vi "setConfiguration.vi"(8 "error in (no error)":errorcluster, 10 "configuration":T1={"exposure_time_s"=nan, "delay_time_s"=nan, "roi"={"x0"=18446744073709551615, "y0"=18446744073709551615, "x1"=18446744073709551615, "y1"=18446744073709551615}, "timestamp_mode"=65535, "pixelrate"=4294967295, "trigger_mode"=65535, "acquire_mode"=65535, "metadata_mode"=65535, "noisefilter_mode"=65535, "binning"={"vert"=65535, "horz"=65535}} {"noisefilter_mode" items=["Undefined"=65535, "OFF"=0, "ON"=1]; "exposure_time_s" format="%#_6f"; "timestamp_mode" items=["Undefined"=65535, "OFF"=0, "Binary"=1, "Binary+ASCII"=2, "ASCII"=3]; "acquire_mode" items=["Undefined"=65535, "auto"=0, "external"=1, "external modulate"=2]; "trigger_mode" items=["Undefined"=65535, "auto sequence"=0, "software trigger"=1, "external exposure start & software trigger"=2, "external exposure control"=3, "external synchronized"=4, "fast external exposure control"=5, "external CDS control"=6, "slow external exposure control"=7, "external synchronized HDSDI"=258]; "metadata_mode" items=["Undefined"=65535, "OFF"=0, "ON"=1]}, 11 "Camera in":refnum<class "Camera.lvclass">) -> (0 "error out":errorcluster, 3 "Camera out":refnum<class "Camera.lvclass">)   [LabVIEW 2020, in "Camera.lvclass"]
doc: "Sets a new coniguration to the camera."
uses:
  Camera.lvclass
  Camera.lvclass/Camera.ctl
  TimingControl.lvlib
  ImageSensor.lvlib
  RecordingControl.lvlib
  GeneralCameraControl.lvlib
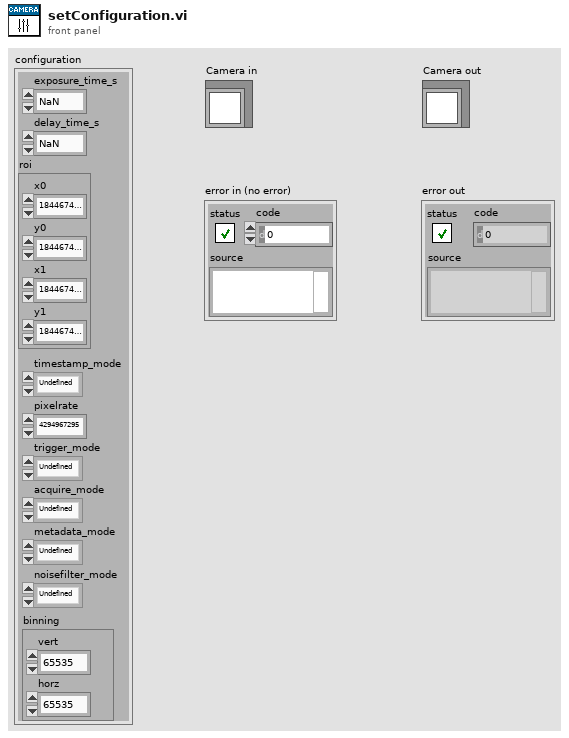
[diagram p1: front panel]
types:
  T1 = cluster{"exposure_time_s":dbl, "delay_time_s":dbl, "roi":cluster{"x0":u64, "y0":u64, "x1":u64, "y1":u64}, "timestamp_mode":u16, "pixelrate":u32, "trigger_mode":u16, "acquire_mode":u16, "metadata_mode":u16, "noisefilter_mode":u16, "binning":cluster{"vert":u16, "horz":u16}}
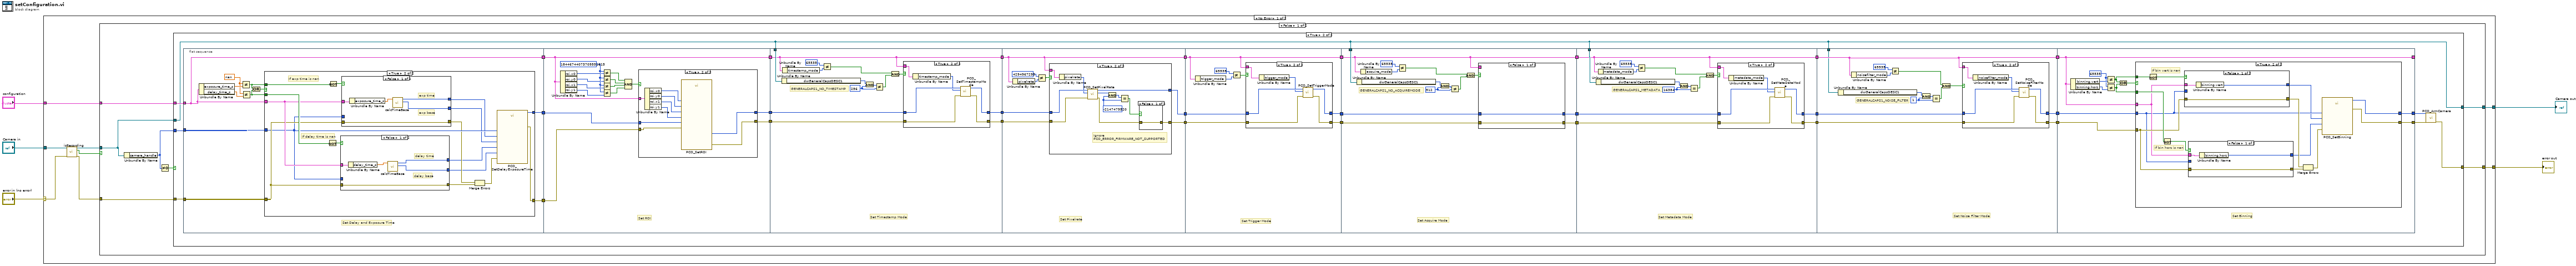
[diagram p0: block diagram]
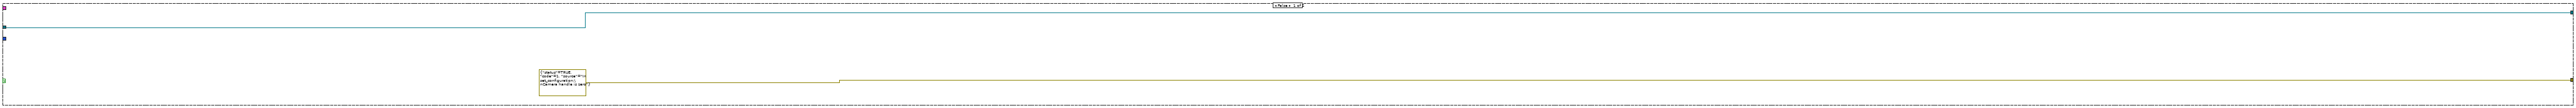
[diagram p2: hidden frame]
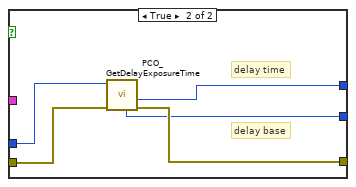
[diagram p4: hidden frame]
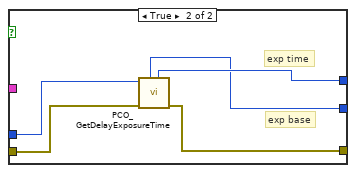
[diagram p5: hidden frame]
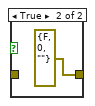
[diagram p9: hidden frame]
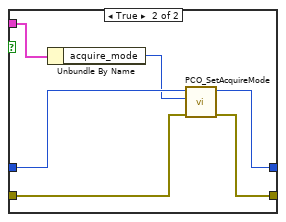
[diagram p11: hidden frame]
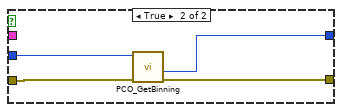
[diagram p15: hidden frame]
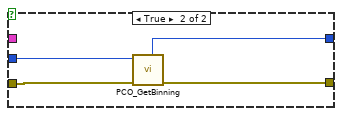
[diagram p16: hidden frame]
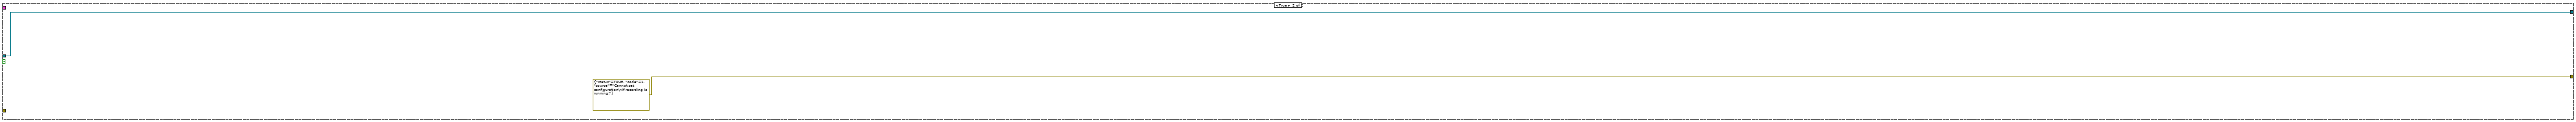
[diagram p17: hidden frame]
diagram:
  n1 = case shown="No Error" "error in (no error)" {
    selector: "error in (no error)" -> [w10 w300]
    tunnel: [w13 w300] -> w4
    tunnel: [w12 w299] -> w2
    tunnel: "Camera in" -> [w11 w299]
    tunnel: "configuration" -> [w6 _]
    frame No Error {
      n2 = call-dynamic "isRecording.vi"("Camera in"=w11, "error in (no error)"=w10) -> ("Camera out"=w7:refnum<class "Camera.lvclass">, "recording"=w9:bool, "error out"=w8:errorcluster)  [unwired: 11 in]
      n3 = case shown="False" w9 {
        tunnel: [w18 errorcluster {"status"=TRUE, "code"=1, "source"="Cannot set configuration\nif recording is running!"} ("error constant")] -> w13
        tunnel: [w17 w297] -> w12
        tunnel: w8 -> [w16 _]
        tunnel: w7 -> [w14 w297]
        tunnel: w6 -> [w15 _]
        frame False {
          n4 = Unbundle By Name(w14) -> ("camera_handle"=w19:u64)
          n5 = Not Equal To 0?(x=w19) -> (x != 0?=w20:bool)
          n6 = case shown="True" w20 {
            tunnel: [errorcluster {"status"=TRUE, "code"=1, "source"="In set_configuration:\nCamera handle is zero"} ("error constant") w24] -> w18
            tunnel: w19 -> [_ w53]
            tunnel: w16 -> [_ w52]
            tunnel: w14 -> [w21 w23]
            tunnel: [w21 w23] -> w17
            tunnel: w15 -> [_ w51]
            frame False {
            }
            frame True {
              n7 = flat-sequence {
                tunnel: w53 -> [w60]
                tunnel: w52 -> [w57]
                tunnel: w51 -> [w56]
                tunnel: [w56] -> w50
                tunnel: [w55] -> w49
                tunnel: [w54] -> w48
                tunnel: w50 -> [w107]
                tunnel: w49 -> [w106]
                tunnel: w48 -> [w105]
                tunnel: [w107] -> w47
                tunnel: [w104] -> w46
                tunnel: [w103] -> w45
                tunnel: w47 -> [w135]
                tunnel: w46 -> [w134]
                tunnel: w45 -> [w133]
                tunnel: w23 -> [w140]
                tunnel: [w135] -> w44
                tunnel: [w132] -> w43
                tunnel: [w131] -> w42
                tunnel: w44 -> [w155]
                tunnel: w43 -> [w154]
                tunnel: w42 -> [w153]
                tunnel: [w155] -> w41
                tunnel: [w152] -> w39
                tunnel: [w151] -> w37
                tunnel: w41 -> [w178]
                tunnel: [w178] -> w40
                tunnel: w39 -> [w177]
                tunnel: [w175] -> w38
                tunnel: w37 -> [w176]
                tunnel: [w174] -> w36
                tunnel: w40 -> [w194]
                tunnel: w38 -> [w197]
                tunnel: w36 -> [w196]
                tunnel: w23 -> [w195]
                tunnel: [w194] -> w35
                tunnel: [w193] -> w34
                tunnel: [w192] -> w33
                tunnel: w35 -> [w214]
                tunnel: w23 -> [w219]
                tunnel: w34 -> [w218]
                tunnel: w33 -> [w217]
                tunnel: [w214] -> w32
                tunnel: [w213] -> w31
                tunnel: [w212] -> w30
                tunnel: w32 -> [w243]
                tunnel: w31 -> [w245]
                tunnel: w30 -> [w244]
                tunnel: [w243] -> w29
                tunnel: [w242] -> w28
                tunnel: [w241] -> w27
                tunnel: w23 -> [w234]
                tunnel: [w258] -> _
                tunnel: w29 -> [w258]
                tunnel: w28 -> [w262]
                tunnel: w27 -> [w261]
                tunnel: [w257] -> w26
                tunnel: [w256] -> w25
                frame #0 {
                  w63 = nan
                  # "Set Delay and Exposure Time"
                  n8 = Unbundle By Name(w56) -> ("exposure_time_s"=w64:dbl, "delay_time_s"=w62:dbl)
                  n9 = Not Equal?(x=w63, y=w64) -> (x != y?=w58:bool)
                  n10 = Not Equal?(x=w63, y=w62) -> (x != y?=w59:bool)
                  n11 = Or(x=w58, y=w59) -> (x .or. y?=w61:bool)
                  n12 = case shown="True" w61 {
                    tunnel: w56 -> [_ w78]
                    tunnel: w60 -> [w66 w76]
                    tunnel: w59 -> [_ w79]
                    tunnel: w58 -> [_ w81]
                    tunnel: w57 -> [w65 w77]
                    tunnel: [w66 w68] -> w55
                    tunnel: [w65 w67] -> w54
                    frame False {
                    }
                    frame True {
                      # "If delay time is nan"
                      # "If exp time is nan"
                      n13 = Not(x=w79) -> (.not. x?=w80:bool)
                      n14 = Not(x=w81) -> (.not. x?=w82:bool)
                      n15 = case shown="False" w80 {
                        tunnel: w76 -> [_ w91]
                        tunnel: w78 -> [w86 _]
                        tunnel: [w85 w89] -> w70
                        tunnel: [w84 w88] -> w69
                        tunnel: w77 -> [w83 w92]
                        tunnel: [w83 w90] -> w73
                        frame False {
                          # "delay base"
                          # "delay time"
                          n16 = Unbundle By Name(w86) -> ("delay_time_s"=w87:dbl)
                          n17 = call "calcTimeBase.vi"("time"=w87) -> ("base_calculated"=w84:u16, "time_calculated"=w85:u32)  [unwired: 9 in]
                        }
                        frame True {
                          # "delay base"
                          # "delay time"
                          n18 = call "PCO_GetDelayExposureTime.vi"("error in (no error)"=w92, "ph"=w91) -> ("error out"=w90:errorcluster, "dwDelay"=w89:u32, "wTimeBaseDelay"=w88:u16)  [unwired: 3 in, 4 out]
                        }
                      }
                      n19 = case shown="False" w82 {
                        tunnel: w76 -> [_ w102]
                        tunnel: w78 -> [w97 _]
                        tunnel: [w95 w99] -> w72
                        tunnel: [w94 w98] -> w71
                        tunnel: w77 -> [w93 w101]
                        tunnel: [w93 w100] -> w74
                        frame False {
                          # "exp base"
                          # "exp time"
                          n20 = Unbundle By Name(w97) -> ("exposure_time_s"=w96:dbl)
                          n21 = call "calcTimeBase.vi"("time"=w96) -> ("base_calculated"=w94:u16, "time_calculated"=w95:u32)  [unwired: 9 in]
                        }
                        frame True {
                          # "exp base"
                          # "exp time"
                          n22 = call "PCO_GetDelayExposureTime.vi"("error in (no error)"=w101, "ph"=w102) -> ("error out"=w100:errorcluster, "dwExposure"=w99:u32, "wTimeBaseExposure"=w98:u16)  [unwired: 3 in, 4 out]
                        }
                      }
                      n23 = Merge Errors(w74, w73) -> (w75:errorcluster)
                      n24 = call "PCO_SetDelayExposureTime.vi"("wTimeBaseExposure"=w71, "wTimeBaseDelay"=w69, "error in (no error)"=w75, "dwExposure"=w72, "dwDelay"=w70, "ph"=w76) -> ("error out"=w67:errorcluster, "ph out"=w68:u64)  [unwired: 3 in, 1 out]
                    }
                  }
                }
                frame #1 {
                  w117 = u64 18446744073709551615
                  # "Set ROI"
                  n25 = Unbundle By Name(w107) -> ("roi.x0"=w116:u64, "roi.y0"=w115:u64, "roi.x1"=w114:u64, "roi.y1"=w113:u64)
                  n26 = Not Equal?(x=w117, y=w116) -> (x != y?=w112:bool)
                  n27 = Not Equal?(x=w117, y=w115) -> (x != y?=w111:bool)
                  n28 = Not Equal?(x=w117, y=w114) -> (x != y?=w110:bool)
                  n29 = Not Equal?(x=w117, y=w113) -> (x != y?=w109:bool)
                  n30 = Compound Arithmetic op=AND(w112, w111, w110, w109) -> (w108:bool)
                  n31 = case shown="True" w108 {
                    tunnel: w107 -> [_ w126]
                    tunnel: w106 -> [w119 w124]
                    tunnel: w105 -> [w118 w125]
                    tunnel: [w119 w128] -> w104
                    tunnel: [w118 w127] -> w103
                    frame False {
                    }
                    frame True {
                      n32 = Unbundle By Name(w126) -> ("roi.x0"=w123:u64, "roi.y0"=w122:u64, "roi.x1"=w121:u64, "roi.y1"=w120:u64)
                      n33 = call "PCO_SetROI.vi"("ph"=w124, "wRoiX0"=w123, "wRoiX1"=w121, "error in (no error)"=w125, "wRoiY0"=w122, "wRoiY1"=w120) -> ("ph out"=w128:u64, "error out"=w127:errorcluster)  [unwired: 7 in, 1 out]
                    }
                  }
                }
                frame #2 {
                  w129 = u32 256 ("camera_description.dwGeneralCapsDESC1")
                  # "Set Timestamp Mode"
                  # "GENERALCAPS1_NO_TIMESTAMP"
                  n34 = Unbundle By Name(w140) -> ("dwGeneralCapsDESC1"=w139:u32)
                  n35 = Unbundle By Name(w135) -> ("timestamp_mode"=w141:u16)
                  n36 = Not Equal?(x=u16 65535 ("timestamp_mode"), y=w141) -> (x != y?=w138:bool)
                  n37 = And(x=w139, y=w129) -> (x .and. y?=w130:u32)
                  n38 = Not Equal?(x=w130, y=w129) -> (x != y?=w137:bool)
                  n39 = And(x=w138, y=w137) -> (x .and. y?=w136:bool)
                  n40 = case shown="True" w136 {
                    tunnel: w135 -> [_ w150]
                    tunnel: w134 -> [w144 w149]
                    tunnel: w133 -> [w143 w148]
                    tunnel: [w144 w146] -> w132
                    tunnel: [w143 w145] -> w131
                    frame False {
                    }
                    frame True {
                      n41 = Unbundle By Name(w150) -> ("timestamp_mode"=w147:u16)
                      n42 = call "PCO_SetTimestampMode.vi"("error in (no error)"=w148, "wTimeStampMode"=w147, "ph"=w149) -> ("error out"=w145:errorcluster, "ph out"=w146:u64)  [unwired: 6 in, 1 out]
                    }
                  }
                }
                frame #3 {
                  # "Set Pixelrate"
                  n43 = Unbundle By Name(w155) -> ("pixelrate"=w158:u32)
                  n44 = Not Equal?(x=u32 4294967295 ("pixelrate"), y=w158) -> (x != y?=w156:bool)
                  n45 = case shown="True" w156 {
                    tunnel: w155 -> [_ w171]
                    tunnel: w154 -> [w160 w170]
                    tunnel: w153 -> [w159 w168]
                    tunnel: [w160 w162] -> w152
                    tunnel: [w159 w161] -> w151
                    frame False {
                    }
                    frame True {
                      w165 = -2147479520 ("ErrorMessage")
                      # "Ignore\nPCO_ERROR_FIRMWARE_NOT_SUPPORTED"
                      n46 = Unbundle By Name(w171) -> ("pixelrate"=w169:u32)
                      n47 = call "PCO_SetPixelRate.vi"("error in (no error)"=w168, "dwPixelRate"=w169, "ph"=w170) -> ("error out"=w163:errorcluster, "ErrorMessage"=w167:i32, "ph out"=w162:u64)  [unwired: 6 in]
                      n48 = And(x=w167, y=w165) -> (x .and. y?=w166:i32)
                      n49 = Equal?(x=w166, y=w165) -> (x = y?=w164:bool)
                      n50 = case shown="False" w164 {
                        tunnel: w163 -> [w172 _]
                        tunnel: [w172 errorcluster {"status"=FALSE, "code"=0, "source"=""} ("error out")] -> w161
                        frame False {
                        }
                        frame True {
                        }
                      }
                    }
                  }
                }
                frame #4 {
                  # "Set Trigger Mode"
                  n51 = Unbundle By Name(w178) -> ("trigger_mode"=w180:u16)
                  n52 = Not Equal?(x=u16 65535 ("timestamp_mode"), y=w180) -> (x != y?=w179:bool)
                  n53 = case shown="True" w179 {
                    tunnel: w178 -> [_ w189]
                    tunnel: w177 -> [w183 w188]
                    tunnel: w176 -> [w182 w187]
                    tunnel: [w183 w185] -> w175
                    tunnel: [w182 w184] -> w174
                    frame False {
                    }
                    frame True {
                      n54 = Unbundle By Name(w189) -> ("trigger_mode"=w186:u16)
                      n55 = call "PCO_SetTriggerMode.vi"("error in (no error)"=w187, "wTriggerMode"=w186, "ph"=w188) -> ("error out"=w184:errorcluster, "ph out"=w185:u64)  [unwired: 6 in, 1 out]
                    }
                  }
                }
                frame #5 {
                  w190 = u32 512 ("camera_description.dwGeneralCapsDESC1")
                  # "Set Acquire Mode"
                  # "GENERALCAPS1_NO_ACQUIREMODE"
                  n56 = Unbundle By Name(w195) -> ("dwGeneralCapsDESC1"=w201:u32)
                  n57 = Unbundle By Name(w194) -> ("acquire_mode"=w202:u16)
                  n58 = Not Equal?(x=u16 65535 ("timestamp_mode"), y=w202) -> (x != y?=w200:bool)
                  n59 = And(x=w201, y=w190) -> (x .and. y?=w191:u32)
                  n60 = Not Equal?(x=w191, y=w190) -> (x != y?=w199:bool)
                  n61 = And(x=w200, y=w199) -> (x .and. y?=w198:bool)
                  n62 = case shown="False" w198 {
                    tunnel: w194 -> [_ w211]
                    tunnel: w197 -> [w205 w210]
                    tunnel: w196 -> [w204 w209]
                    tunnel: [w205 w207] -> w193
                    tunnel: [w204 w206] -> w192
                    frame False {
                    }
                    frame True {
                      n63 = Unbundle By Name(w211) -> ("acquire_mode"=w208:u16)
                      n64 = call "PCO_SetAcquireMode.vi"("error in (no error)"=w209, "wAcquMode"=w208, "ph"=w210) -> ("error out"=w206:errorcluster, "ph out"=w207:u64)  [unwired: 6 in, 1 out]
                    }
                  }
                }
                frame #6 {
                  w215 = u32 16384 ("camera_description.dwGeneralCapsDESC1")
                  # "Set Metadata Mode"
                  # "GENERALCAPS1_METADATA"
                  n65 = Unbundle By Name(w219) -> ("dwGeneralCapsDESC1"=w223:u32)
                  n66 = Unbundle By Name(w214) -> ("metadata_mode"=w224:u16)
                  n67 = Not Equal?(x=u16 65535 ("timestamp_mode"), y=w224) -> (x != y?=w222:bool)
                  n68 = And(x=w223, y=w215) -> (x .and. y?=w216:u32)
                  n69 = Equal?(x=w216, y=w215) -> (x = y?=w221:bool)
                  n70 = And(x=w222, y=w221) -> (x .and. y?=w220:bool)
                  n71 = case shown="True" w220 {
                    tunnel: w214 -> [_ w233]
                    tunnel: w218 -> [w227 w232]
                    tunnel: w217 -> [w226 w231]
                    tunnel: [w227 w229] -> w213
                    tunnel: [w226 w228] -> w212
                    frame False {
                    }
                    frame True {
                      n72 = Unbundle By Name(w233) -> ("metadata_mode"=w230:u16)
                      n73 = call "PCO_SetMetaDataMode.vi"("error in (no error)"=w231, "wMetaDataMode"=w230, "ph"=w232) -> ("error out"=w228:errorcluster, "ph out"=w229:u64)  [unwired: 4 in, 3 out]
                    }
                  }
                }
                frame #7 {
                  w238 = u32 1 ("camera_description.dwGeneralCapsDESC1")
                  # "GENERALCAPS1_NOISE_FILTER"
                  # "Set Noise Filter Mode"
                  n74 = Unbundle By Name(w234) -> ("dwGeneralCapsDESC1"=w240:u32)
                  n75 = Unbundle By Name(w243) -> ("noisefilter_mode"=w246:u16)
                  n76 = Not Equal?(x=u16 65535 ("timestamp_mode"), y=w246) -> (x != y?=w237:bool)
                  n77 = And(x=w240, y=w238) -> (x .and. y?=w239:u32)
                  n78 = Equal?(x=w239, y=w238) -> (x = y?=w236:bool)
                  n79 = And(x=w237, y=w236) -> (x .and. y?=w235:bool)
                  n80 = case shown="True" w235 {
                    tunnel: w243 -> [_ w255]
                    tunnel: w245 -> [w249 w254]
                    tunnel: w244 -> [w248 w253]
                    tunnel: [w249 w251] -> w242
                    tunnel: [w248 w250] -> w241
                    frame False {
                    }
                    frame True {
                      n81 = Unbundle By Name(w255) -> ("noisefilter_mode"=w252:u16)
                      n82 = call "PCO_SetNoiseFilterMode.vi"("error in (no error)"=w253, "wNoiseFilterMode"=w252, "ph"=w254) -> ("error out"=w250:errorcluster, "ph out"=w251:u64)  [unwired: 6 in, 1 out]
                    }
                  }
                }
                frame #8 {
                  w264 = u16 65535 ("timestamp_mode")
                  # "Set Binning"
                  n83 = Unbundle By Name(w258) -> ("binning.vert"=w266:u16, "binning.horz"=w265:u16)
                  n84 = Not Equal?(x=w264, y=w266) -> (x != y?=w260:bool)
                  n85 = Not Equal?(x=w264, y=w265) -> (x != y?=w259:bool)
                  n86 = Or(x=w260, y=w259) -> (x .or. y?=w263:bool)
                  n87 = case shown="True" w263 {
                    tunnel: w262 -> [w268 w272]
                    tunnel: w261 -> [w267 w278]
                    tunnel: [w268 w269] -> w257
                    tunnel: [w267 w270] -> w256
                    tunnel: w260 -> [_ w282]
                    tunnel: w259 -> [_ w281]
                    tunnel: w258 -> [_ w277]
                    frame False {
                    }
                    frame True {
                      # "If bin horz is nan"
                      # "If bin vert is nan"
                      n88 = Not(x=w282) -> (.not. x?=w280:bool)
                      n89 = Not(x=w281) -> (.not. x?=w279:bool)
                      n90 = case shown="False" w280 {
                        tunnel: w277 -> [w292 _]
                        tunnel: [w291 w294] -> w271
                        tunnel: w272 -> [_ w296]
                        tunnel: w278 -> [w290 w295]
                        tunnel: [w290 w293] -> w275
                        frame False {
                          n91 = Unbundle By Name(w292) -> ("binning.vert"=w291:u16)
                        }
                        frame True {
                          n92 = call "PCO_GetBinning.vi"("error in (no error)"=w295, "ph"=w296) -> ("error out"=w293:errorcluster, "wBinVert"=w294:u16)  [unwired: 5 in, 3 out]
                        }
                      }
                      n93 = case shown="False" w279 {
                        tunnel: w277 -> [w285 _]
                        tunnel: [w284 w286] -> w273
                        tunnel: w272 -> [_ w289]
                        tunnel: w278 -> [w283 w288]
                        tunnel: [w283 w287] -> w276
                        frame False {
                          n94 = Unbundle By Name(w285) -> ("binning.horz"=w284:u16)
                        }
                        frame True {
                          n95 = call "PCO_GetBinning.vi"("error in (no error)"=w288, "ph"=w289) -> ("error out"=w287:errorcluster, "wBinHorz"=w286:u16)  [unwired: 5 in, 3 out]
                        }
                      }
                      n96 = Merge Errors(w275, w276) -> (w274:errorcluster)
                      n97 = call "PCO_SetBinning.vi"("error in (no error)"=w274, "wBinVert"=w271, "wBinHorz"=w273, "ph"=w272) -> ("error out"=w270:errorcluster, "ph out"=w269:u64)  [unwired: 5 in, 1 out]
                    }
                  }
                }
              }
              n98 = call "PCO_ArmCamera.vi"("error in (no error)"=w25, "ph"=w26) -> ("error out"=w24:errorcluster)  [unwired: 7 in, 2 out]
            }
          }
        }
        frame True {
        }
      }
    }
    frame Error {
    }
  }
  "error out" <- w4
  "Camera out" <- w2
